vi "CallBack_MouseUp.vi"(4 "Data":T1, 5 "Event Data":cluster{"sender":refnum<k24>, "e":refnum<k24>}, 6 "Control Ref":refnum<k24>, 7 "Event Common Data":T2) -> ()   [LabVIEW 2020, in "LcPictureBox.lvclass"]
uses:
  LcPictureBox.lvclass
  System.Windows.Forms
  CallBacks/MouseInfo.ctl
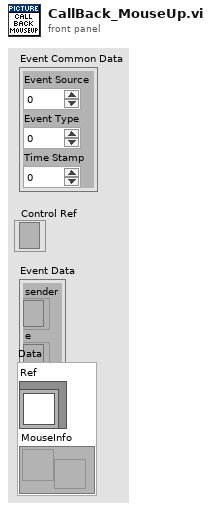
[diagram p1: front panel]
types:
  T1 = cluster{"Ref":refnum<class "LcPictureBox.lvclass">, "MouseInfo":refnum<user-event>}
  T2 = cluster{"Event Source":i32, "Event Type":u32, "Time Stamp":u32}
  T3 = typedef "LcPictureBox.lvclass/MouseInfo.ctl" = cluster{"X":i32, "Y":i32, "Button":i32}
  T4 = typedef "LcPictureBox.lvclass/ObjectAttributes.ctl" = cluster{"PictureBox":refnum<k24>, "ImageSize":cluster{"Width":i32, "Height":i32}, "PenMemory":map{cluster{"Alpha(100%)":dbl, "Color(Black)":u32, "Pen(Width=1, Solid)":T5}, refnum<k24>}, "GraphicsRef":refnum<k24>, "BrushMemory":map{cluster{"Alpha(100%)":dbl, "Color(Black)":u32}, refnum<k24>}, "Images":refnum<k24>[], "ImageIndex":i32, "BgColor(None)":u32, "LoadedImages":map{string, cluster{"ImageOut":refnum<k24>, "ImageSize":cluster{"Width":i32, "Height":i32}}}, "ColorsMemory":map{cluster{"Alpha(100%)":dbl, "Color(Black)":u32}, refnum<k24>}, "CacheSize":i32, "PictureBoxActiveXReference":refnum<vi>, "Scale":sgl, "Offset":cluster{"x":sgl, "y":sgl}, "zoom_center":cluster{"X":i32, "Y":i32}, "ImagesCreated":refnum<k24>[]}
  T5 = typedef "LcPictureBox.lvclass/Pen.ctl" = cluster{"Width":u16, "Style":enum32{"Solid", "Dash", "Dot", "DashDot", "DashDotDot"}}
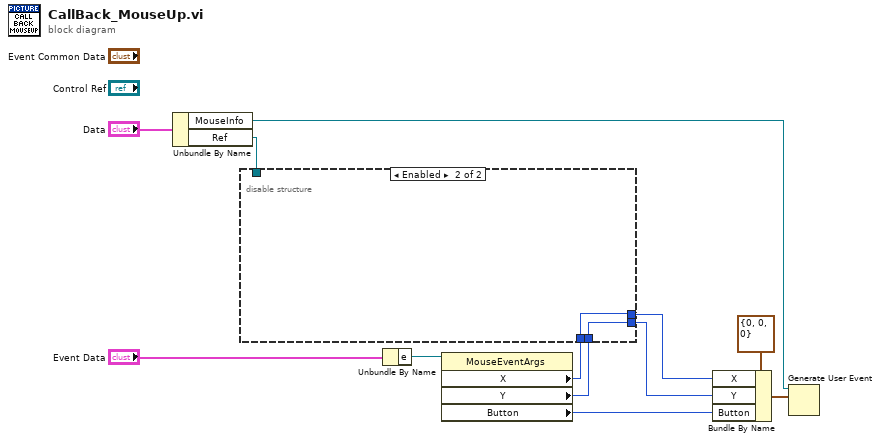
[diagram p0: block diagram]
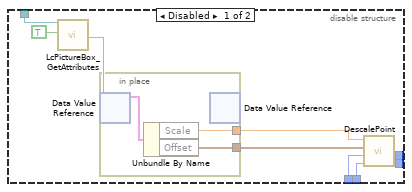
[diagram p2: hidden frame]
diagram:
  n1 = Unbundle By Name("Data") -> ("MouseInfo"=w3:refnum<user-event>, "Ref"=w7:refnum<class "LcPictureBox.lvclass">)
  n2 = Unbundle By Name("Event Data") -> ("e"=w12:refnum<k24>)
  n3 = property class="MouseEventArgs"(reference=w12) -> ("X"=w2:i32, "Y"=w1:i32, "Button"=w9:i32)  [unwired: 1 in, 2 out]
  n4 = disable-structure shown="Enabled" {
    disable-tunnel: w7 -> [w21 _]
    disable-tunnel: [w16 w26] -> w6
    disable-tunnel: [w15 w25] -> w5
    disable-tunnel: w2 -> [w14 w26]
    disable-tunnel: w1 -> [w13 w25]
    frame Disabled {
      n5 = call "LcPictureBox_GetAttributes.vi"("reference in"=w21, "OnlyGetDvrReference(False)"=TRUE) -> ("DataRef"=w19:refnum<data-value>)  [unwired: 14 in, 3 out]
      n6 = in-place {
        in-place-border: [w23] -> w18
        in-place-border: [w22] -> w17
        n7 = in-place-dvr #1(w19) -> (w24:T4)  [unwired: 1 out]
        n8 = Unbundle By Name(w24) -> ("Scale"=w22:sgl, "Offset"=w23:cluster{"x":sgl, "y":sgl})
        n9 = in-place-dvr #1() -> ()  [unwired: 1 in, 2 out]
      }
      n10 = call "DescalePoint.vi"("Y"=w13, "X"=w14, "Offset"=w18, "Scale"=w17) -> ("Y-Out"=w15:sgl, "X-Out"=w16:sgl)  [unwired: 6 in]
    }
    frame Enabled {
    }
  }
  n11 = Bundle By Name(cluster=T3 {"X"=0, "Y"=0, "Button"=0} ("event data"), "X"=w6, "Y"=w5, "Button"=w9) -> (w10:T3)
  n12 = Generate User Event(user event=w3, event data cluster=w10) -> ()  [unwired: 2 in, 2 out]
